vi "Configure Chevelle JESD Rx.vi"(0 "rx baseband session in":T1={"3630 session"={"VISA resource name"="", "Address Space"=1, "window_offset"=0, "register_addresses"={"MM based Registers"={"Revision"=0, "OldestCompatRev"=0, "signature"=0, "scratch"=0, "LedControl"=0, "BoardHwRev"=0, "BoardControl"=0, "ThermalStatus"=0, "BasebandStatus"=0, "BasebandControl"=0, "BasebandAuxSetup"=0, "BasebandAuxStatus"=0, "LmkSyncOutSetup"=0, " AdcSyncOutSetup"=0, " InjSyncOutSetup"=0, " PxiTrig0OutSetup"=0, " PxiTrig1OutSetup"=0, " PxiTrig2OutSetup"=0, " PxiTrig3OutSetup"=0, " PxiTrig4OutSetup"=0, " PxiTrig5OutSetup"=0, " PxiTrig6OutSetup"=0, " PxiTrig7OutSetup"=0}, "CPLD based Registers"={"SlaveSignature"=0, "SlaveRevision"=0, "SlaveOldestCompatRev"=0, "SlaveScratch"=0, "SlaveSetup"=0, "SlaveStatus"=0, "IDacReg_offset"=0, "LMKRegGrp0_offset"=0, "QDacReg_offset"=0, "BrdTempSensorVal"=0, "TempSensorPowerDown"=0, "GPIOReg_offset"=0, "IAdcReg_offset"=0, "QAdcReg_offset"=0, "LMKRegGrp1_offset"=0, "QadcTempSensorVal"=0, "IadcTempSensorVal"=0, "RevisionReg"=0, "VcxoReg"=0, "CpldStatusReg"=0, "PowerReg"=0, "VBiasEnReg"=0, "ExtRefOeReg"=0, "QdacCtrlReg"=0, "QdacStatusReg"=0, "IdacCtrlReg"=0, "IdacStatusReg"=0, "QdacJtagIn"=0, "QdacJtagOut"=0, "IdacJtagIn"=0, "IdacJtagOut"=0, "IqDcSetupReg"=0, "QadcStatusReg"=0, "IadcStatusReg"=0, "BrdSetupReg"=0, "IqDcRevisionReg"=0, "PllStatusReg"=0, "EndpointScratchReg"=0, "AdcSyncCfgReg"=0, "IqCardOpampReg"=0}, "CPLD Register Offset"=0, "MM  Register Offset"=0, " PxiTrig0OutSetup"=0}, "required_MM_fpga_version"={"signature"=0, "hardware"=0, "current revision"=0, "oldest revision"=0}, "CPLD Oldest Compat Version "={"hardware"=0, "CPLD firmware"=0}, "MM_FPGA_image_location"="", "is_init"=FALSE, "card_type"=enum."ADC", "DacLmkConfigFileName"="", "AdcLmkConfigFileName"="", "AdcConfigFileName"="", "DacConfigFileName_RevA"="", "DacConfigFileName_RevB"="", "Mulde hardware revision"=0, "bypass DAC PLL\n"=FALSE, "IQ Card Revision"=enum."RevA", "board capability"={"baseband sync"=enum."no baseband sync"}}, "7902 reference"=refnum} {"3630 session"."Address Space" items=["VXI/VME A16"=1, "VXI/VME A24"=2, "VXI/VME A32"=3, "VXI/VME A64"=4, "PXI Memory Allocations"=9, "PXI Configuration"=10, "PXI BAR0"=11, "PXI BAR1"=12, "PXI BAR2"=13, "PXI BAR3"=14, "PXI BAR4"=15, "PXI BAR5"=16]}, 11 "error in":errorcluster) -> (4 "rx baseband session":T1={"3630 session"={"VISA resource name"="", "Address Space"=1, "window_offset"=0, "register_addresses"={"MM based Registers"={"Revision"=0, "OldestCompatRev"=0, "signature"=0, "scratch"=0, "LedControl"=0, "BoardHwRev"=0, "BoardControl"=0, "ThermalStatus"=0, "BasebandStatus"=0, "BasebandControl"=0, "BasebandAuxSetup"=0, "BasebandAuxStatus"=0, "LmkSyncOutSetup"=0, " AdcSyncOutSetup"=0, " InjSyncOutSetup"=0, " PxiTrig0OutSetup"=0, " PxiTrig1OutSetup"=0, " PxiTrig2OutSetup"=0, " PxiTrig3OutSetup"=0, " PxiTrig4OutSetup"=0, " PxiTrig5OutSetup"=0, " PxiTrig6OutSetup"=0, " PxiTrig7OutSetup"=0}, "CPLD based Registers"={"SlaveSignature"=0, "SlaveRevision"=0, "SlaveOldestCompatRev"=0, "SlaveScratch"=0, "SlaveSetup"=0, "SlaveStatus"=0, "IDacReg_offset"=0, "LMKRegGrp0_offset"=0, "QDacReg_offset"=0, "BrdTempSensorVal"=0, "TempSensorPowerDown"=0, "GPIOReg_offset"=0, "IAdcReg_offset"=0, "QAdcReg_offset"=0, "LMKRegGrp1_offset"=0, "QadcTempSensorVal"=0, "IadcTempSensorVal"=0, "RevisionReg"=0, "VcxoReg"=0, "CpldStatusReg"=0, "PowerReg"=0, "VBiasEnReg"=0, "ExtRefOeReg"=0, "QdacCtrlReg"=0, "QdacStatusReg"=0, "IdacCtrlReg"=0, "IdacStatusReg"=0, "QdacJtagIn"=0, "QdacJtagOut"=0, "IdacJtagIn"=0, "IdacJtagOut"=0, "IqDcSetupReg"=0, "QadcStatusReg"=0, "IadcStatusReg"=0, "BrdSetupReg"=0, "IqDcRevisionReg"=0, "PllStatusReg"=0, "EndpointScratchReg"=0, "AdcSyncCfgReg"=0, "IqCardOpampReg"=0}, "CPLD Register Offset"=0, "MM  Register Offset"=0, " PxiTrig0OutSetup"=0}, "required_MM_fpga_version"={"signature"=0, "hardware"=0, "current revision"=0, "oldest revision"=0}, "CPLD Oldest Compat Version "={"hardware"=0, "CPLD firmware"=0}, "MM_FPGA_image_location"="", "is_init"=FALSE, "card_type"=enum."ADC", "DacLmkConfigFileName"="", "AdcLmkConfigFileName"="", "AdcConfigFileName"="", "DacConfigFileName_RevA"="", "DacConfigFileName_RevB"="", "Mulde hardware revision"=0, "bypass DAC PLL\n"=FALSE, "IQ Card Revision"=enum."RevA", "board capability"={"baseband sync"=enum."no baseband sync"}}, "7902 reference"=refnum} {"3630 session"."Address Space" items=["VXI/VME A16"=1, "VXI/VME A24"=2, "VXI/VME A32"=3, "VXI/VME A64"=4, "PXI Memory Allocations"=9, "PXI Configuration"=10, "PXI BAR0"=11, "PXI BAR1"=12, "PXI BAR2"=13, "PXI BAR3"=14, "PXI BAR4"=15, "PXI BAR5"=16]}, 15 "error out":errorcluster)   [LabVIEW 2019]
uses:
  TypeDefs/Rx Baseband Session.ctl
  <instrlib>/niMmWave/ni3610 and ni3630/controls/public/Main Settings.ctl
  <vilib>/Instr/_visa.llb/VISA Register Access Address Space.ctl
  <instrlib>/niMmWave/ni3610 and ni3630/controls/public/Register Adresses.ctl
  <instrlib>/niMmWave/ni3610 and ni3630/controls/public/Base Card Type.ctl
  <instrlib>/niMmWave/ni3610 and ni3630/controls/private/IQ Card Revision.ctl
  <instrlib>/niMmWave/ni3610 and ni3630/controls/public/Board Capability.ctl
  TypeDefs/Blank FPGA Reference.ctl
  TypeDefs/RX FPGA Reference.ctl
  <vilib>/rvi/errors/niLvFpgaAdjustHostInterfaceError.vi
  <vilib>/rvi/interface/nirviReadWriteControl/nirviReadWriteControl.xnode
  <vilib>/rvi/interface/Simulation/niFpgaSimulationCallBeginRW.vi
  NiFpgaLv.dll
  <instrlib>/niMmWave/ni3610 and ni3630/ni3610_and_ni3630_Driver_Lib.lvlib
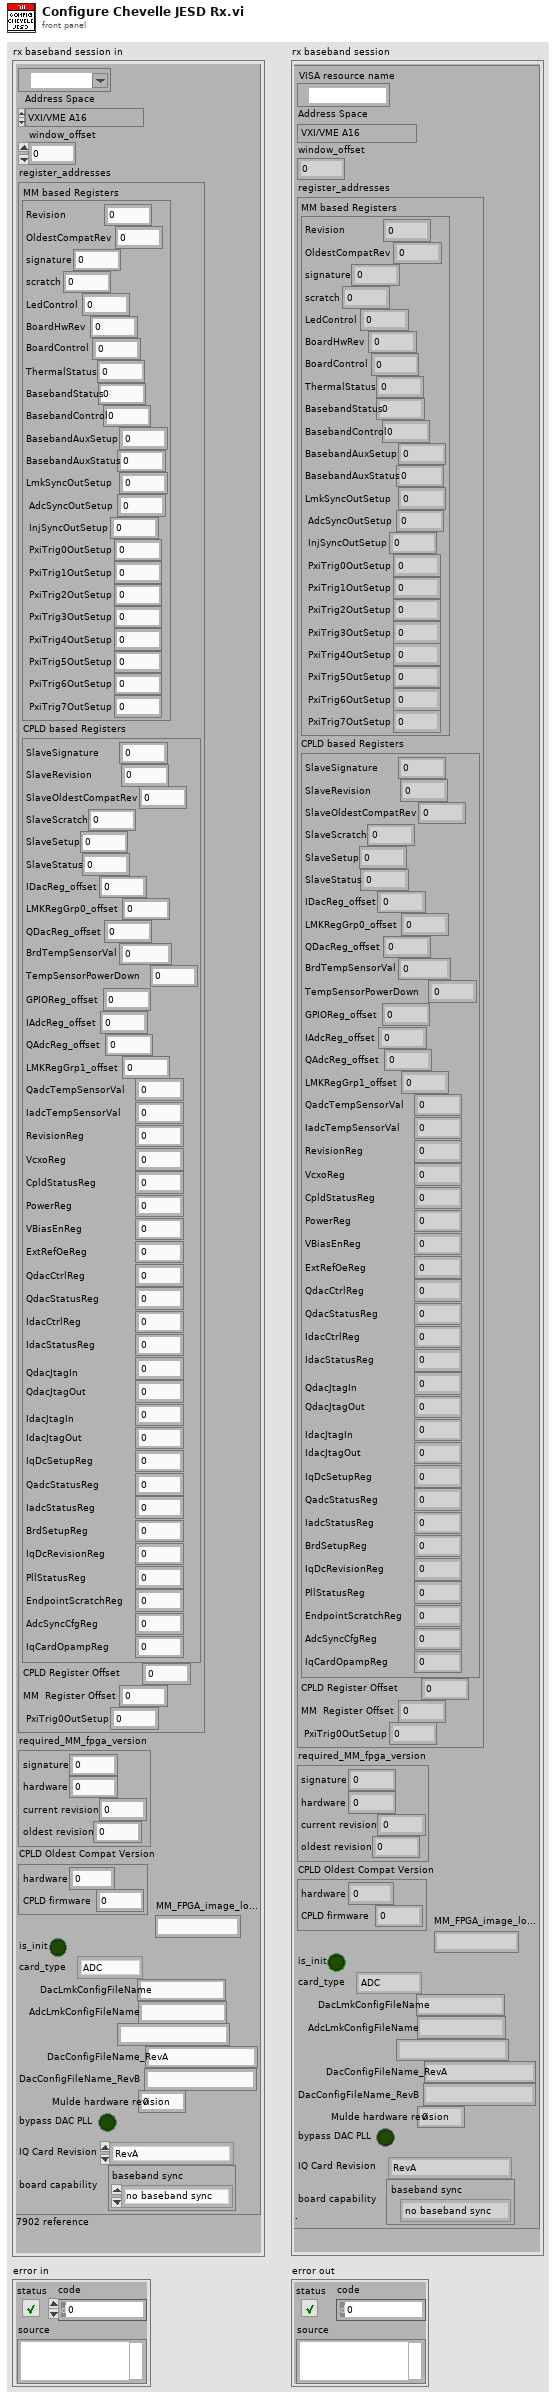
[diagram p1: front panel]
types:
  T1 = typedef "Rx Baseband Session.ctl" = cluster{"3630 session":T2, "7902 reference":T8}
  T2 = typedef "ni3610_and_ni3630_Driver_Lib.lvlib/Main Settings.ctl" = cluster{"VISA resource name":refnum<visa-resource-name>, "Address Space":T3, "window_offset":u32, "register_addresses":T4, "required_MM_fpga_version":cluster{"signature":u32, "hardware":u32, "current revision":u32, "oldest revision":u32}, "CPLD Oldest Compat Version ":cluster{"hardware":u32, "CPLD firmware":u32}, "MM_FPGA_image_location":string, "is_init":bool, "card_type":T5, "DacLmkConfigFileName":string, "AdcLmkConfigFileName":string, "AdcConfigFileName":string, "DacConfigFileName_RevA":string, "DacConfigFileName_RevB":string, "Mulde hardware revision":u8, "bypass DAC PLL\n":bool, "IQ Card Revision":T6, "board capability":T7}
  T3 = typedef "VISA Register Access Address Space.ctl" = u16
  T4 = typedef "ni3610_and_ni3630_Driver_Lib.lvlib/Register Adresses.ctl" = cluster{"MM based Registers":cluster{"Revision":u32, "OldestCompatRev":u32, "signature":u32, "scratch":u32, "LedControl":u32, "BoardHwRev":u32, "BoardControl":u32, "ThermalStatus":u32, "BasebandStatus":u32, "BasebandControl":u32, "BasebandAuxSetup":u32, "BasebandAuxStatus":u32, "LmkSyncOutSetup":u32, " AdcSyncOutSetup":u32, " InjSyncOutSetup":u32, " PxiTrig0OutSetup":u32, " PxiTrig1OutSetup":u32, " PxiTrig2OutSetup":u32, " PxiTrig3OutSetup":u32, " PxiTrig4OutSetup":u32, " PxiTrig5OutSetup":u32, " PxiTrig6OutSetup":u32, " PxiTrig7OutSetup":u32}, "CPLD based Registers":cluster{"SlaveSignature":u32, "SlaveRevision":u32, "SlaveOldestCompatRev":u32, "SlaveScratch":u32, "SlaveSetup":u32, "SlaveStatus":u32, "IDacReg_offset":u32, "LMKRegGrp0_offset":u32, "QDacReg_offset":u32, "BrdTempSensorVal":u32, "TempSensorPowerDown":u32, "GPIOReg_offset":u32, "IAdcReg_offset":u32, "QAdcReg_offset":u32, "LMKRegGrp1_offset":u32, "QadcTempSensorVal":u32, "IadcTempSensorVal":u32, "RevisionReg":u32, "VcxoReg":u32, "CpldStatusReg":u32, "PowerReg":u32, "VBiasEnReg":u32, "ExtRefOeReg":u32, "QdacCtrlReg":u32, "QdacStatusReg":u32, "IdacCtrlReg":u32, "IdacStatusReg":u32, "QdacJtagIn":u32, "QdacJtagOut":u32, "IdacJtagIn":u32, "IdacJtagOut":u32, "IqDcSetupReg":u32, "QadcStatusReg":u32, "IadcStatusReg":u32, "BrdSetupReg":u32, "IqDcRevisionReg":u32, "PllStatusReg":u32, "EndpointScratchReg":u32, "AdcSyncCfgReg":u32, "IqCardOpampReg":u32}, "CPLD Register Offset":u32, "MM  Register Offset":u32, " PxiTrig0OutSetup":u32}
  T5 = typedef "ni3610_and_ni3630_Driver_Lib.lvlib/Base Card Type.ctl" = enum16{"unspecified", "ADC", "DAC"}
  T6 = typedef "ni3610_and_ni3630_Driver_Lib.lvlib/IQ Card Revision.ctl" = enum16{"RevA", "RevB", "RevC", "RevD"}
  T7 = typedef "ni3610_and_ni3630_Driver_Lib.lvlib/Board Capability.ctl" = cluster{"baseband sync":enum16{"no baseband sync", "baseband sync"}}
  T8 = typedef "Blank FPGA Reference.ctl" = refnum<k20>
  T9 = typedef "RX FPGA Reference.ctl" = refnum<k20>
  T10 = cluster{"gtx active":bool, "jesd active":bool, "lane sync req":bool, "lanes synced":bool, "lanes aligned":bool, "qpll locked":bool, "qpll ref lost":bool, "k-char error":bool, "lane alignment error":bool, "8b10b error":bool, "8b10b disparity error":bool, "buffer overflow":bool, "buffer underflow":bool, "buffer ready":bool, "mgt ref clocks locked":bool, "mgt ref clock valid":bool, "config complete":bool}
  T11 = cluster{"gtx enable":bool, "jesd enable":bool, "sw sync":bool, "buffer enable":bool, "clock enable":bool, "trig5 output enable":bool, "trig5 invert":bool}
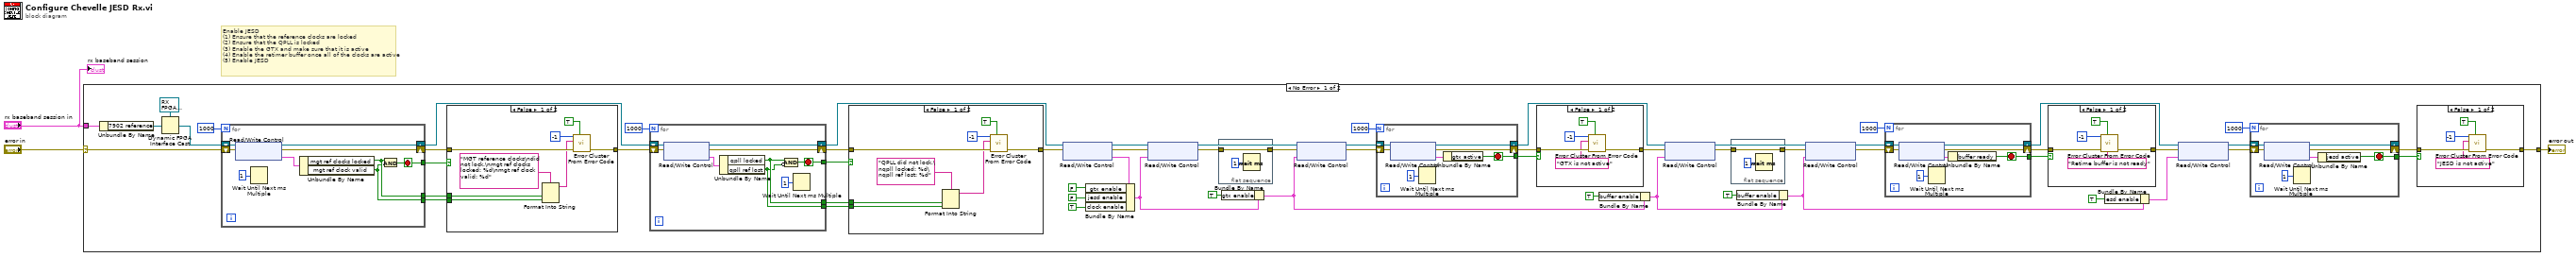
[diagram p0: block diagram]
diagram:
  # "Enable JESD\n(1) Ensure that the reference clocks are locked\n(2) Ensure that the QPLL is locked\n(3) Enable the GTX and make sure that it is active\n(4) Enable the retimer buffer once all of the clocks are active\n(5) Enable JESD"
  n1 = case shown="No Error" "error in" {
    selector: "error in" -> [w55 w143]
    tunnel: "rx baseband session in" -> [w34 _]
    tunnel: [w36 w143] -> w3
    frame No Error {
      n2 = Unbundle By Name(w34) -> ("7902 reference"=w35:T8)
      n3 = Dynamic FPGA Interface Cast(Session In=T9 refnum ("fpga reference"), Type=w35) -> (Session Out=w54:T9)
      n4 = for {
        N: 1000 -> [_]
        shift-right: [w76] -> w57
        shift-left: w54 -> [w74]
        shift-right: [w75] -> w59
        shift-left: w55 -> [w73]
        tunnel: [w71] -> w58
        tunnel: [w69] -> w7
        tunnel: [w68] -> w6
        stop <- w71 stop-if-true
        n5 = xnode "Read/Write Control"("FPGA VI Reference In"=w74, "error in"=w73) -> ("FPGA VI Reference Out"=w76:T9, "error out"=w75:errorcluster, "rxjesd.status"=w70:T10)
        n6 = Wait Until Next ms Multiple(millisecond multiple=u32 1) -> ()  [unwired: 1 out]
        n7 = Unbundle By Name(w70) -> ("mgt ref clocks locked"=w69:bool, "mgt ref clock valid"=w68:bool)
        n8 = Compound Arithmetic op=AND(w69, w68) -> (w71:bool)
      }
      n9 = case shown="False" w58 {
        tunnel: w59 -> [w84 w85]
        tunnel: [w83 w85] -> w56
        tunnel: w7 -> [w79 _]
        tunnel: w6 -> [w78 _]
        frame False {
          n10 = Format Into String(format string="MGT reference clocks\ndid not lock.\nmgt ref clocks locked: %d\nmgt ref clock valid: %d", w79, w78) -> (resulting string=w77:string)  [unwired: 2 in, 1 out]
          n11 = call <vilib>:"Error Cluster From Error Code.vi"("show call chain? (False)"=TRUE ("is warning? (False)"), "error in (no error)"=w84, "error message (\"\")"=w77, "error code (0)"=-1) -> ("error out"=w83:errorcluster)  [unwired: 5 in]
        }
        frame True {
        }
      }
      n12 = for {
        N: 1000 -> [_]
        shift-right: [w94] -> w12
        shift-left: w57 -> [w92]
        shift-right: [w93] -> w50
        shift-left: w56 -> [w91]
        tunnel: [w89] -> w51
        tunnel: [w87] -> w5
        tunnel: [w86] -> w4
        stop <- w89 stop-if-true
        n13 = xnode "Read/Write Control"("FPGA VI Reference In"=w92, "error in"=w91) -> ("FPGA VI Reference Out"=w94:T9, "error out"=w93:errorcluster, "rxjesd.status"=w88:T10)
        n14 = Unbundle By Name(w88) -> ("qpll locked"=w87:bool, "qpll ref lost"=w86:bool)
        n15 = Compound Arithmetic op=AND(w87, invert w86) -> (w89:bool)
        n16 = Wait Until Next ms Multiple(millisecond multiple=u32 1) -> ()  [unwired: 1 out]
      }
      n17 = case shown="False" w51 {
        tunnel: w50 -> [w102 w103]
        tunnel: [w101 w103] -> w13
        tunnel: w5 -> [w96 _]
        tunnel: w4 -> [w95 _]
        frame False {
          n18 = Format Into String(format string="QPLL did not lock.\nqpll locked: %d\nqpll ref lost: %d", w96, w95) -> (resulting string=w97:string)  [unwired: 2 in, 1 out]
          n19 = call <vilib>:"Error Cluster From Error Code.vi"("show call chain? (False)"=TRUE ("is warning? (False)"), "error in (no error)"=w102, "error message (\"\")"=w97, "error code (0)"=-1) -> ("error out"=w101:errorcluster)  [unwired: 5 in]
        }
        frame True {
        }
      }
      n20 = xnode "Read/Write Control"("FPGA VI Reference In"=w12, "error in"=w13) -> ("FPGA VI Reference Out"=w11:T9, "error out"=w14:errorcluster, "rxjesd.control"=w31:T11)
      n21 = Bundle By Name(cluster=w31, "gtx enable"=FALSE ("rxjesd.gtx enable"), "jesd enable"=FALSE ("rxjesd.jesd enable"), "clock enable"=TRUE ("clk enable")) -> (w17:T11)
      n22 = xnode "Read/Write Control"("FPGA VI Reference In"=w11, "error in"=w14, "rxjesd.control"=w17) -> ("FPGA VI Reference Out"=w53:T9, "error out"=w62:errorcluster)
      n23 = flat-sequence {
        tunnel: w62 -> [w66]
        tunnel: [w66] -> w52
        frame #0 {
          n24 = Wait (ms)(milliseconds to wait=u32 1) -> ()  [unwired: 1 out]
        }
      }
      n25 = Bundle By Name(cluster=w17, "gtx enable"=TRUE) -> (w8:T11)
      n26 = xnode "Read/Write Control"("FPGA VI Reference In"=w53, "error in"=w52, "rxjesd.control"=w8) -> ("FPGA VI Reference Out"=w47:T9, "error out"=w48:errorcluster)
      n27 = for {
        N: 1000 -> [_]
        shift-right: [w110] -> w33
        shift-left: w47 -> [w108]
        shift-right: [w109] -> w46
        shift-left: w48 -> [w107]
        tunnel: [w104] -> w45
        stop <- w104 stop-if-true
        n28 = xnode "Read/Write Control"("FPGA VI Reference In"=w108, "error in"=w107) -> ("FPGA VI Reference Out"=w110:T9, "error out"=w109:errorcluster, "rxjesd.status"=w105:T10)
        n29 = Wait Until Next ms Multiple(millisecond multiple=u32 1) -> ()  [unwired: 1 out]
        n30 = Unbundle By Name(w105) -> ("gtx active"=w104:bool)
      }
      n31 = case shown="False" w45 {
        tunnel: w46 -> [w115 w116]
        tunnel: [w114 w116] -> w32
        frame False {
          n32 = call <vilib>:"Error Cluster From Error Code.vi"("show call chain? (False)"=TRUE ("is warning? (False)"), "error in (no error)"=w115, "error message (\"\")"="GTX is not active" ("source"), "error code (0)"=-1) -> ("error out"=w114:errorcluster)  [unwired: 5 in]
        }
        frame True {
        }
      }
      n33 = Bundle By Name(cluster=w8, "buffer enable"=TRUE ("gtx enable")) -> (w16:T11)
      n34 = xnode "Read/Write Control"("FPGA VI Reference In"=w33, "error in"=w32, "rxjesd.control"=w16) -> ("FPGA VI Reference Out"=w22:T9, "error out"=w23:errorcluster)
      n35 = flat-sequence {
        tunnel: w23 -> [w64]
        tunnel: [w64] -> w19
        frame #0 {
          n36 = Wait (ms)(milliseconds to wait=u32 1) -> ()  [unwired: 1 out]
        }
      }
      n37 = Bundle By Name(cluster=w16, "buffer enable"=TRUE ("gtx enable")) -> (w15:T11)
      n38 = xnode "Read/Write Control"("FPGA VI Reference In"=w22, "error in"=w19, "rxjesd.control"=w15) -> ("FPGA VI Reference Out"=w21:T9, "error out"=w20:errorcluster)
      n39 = for {
        N: 1000 -> [_]
        shift-right: [w123] -> w10
        shift-left: w21 -> [w121]
        shift-right: [w122] -> w9
        shift-left: w20 -> [w120]
        tunnel: [w117] -> w43
        stop <- w117 stop-if-true
        n40 = xnode "Read/Write Control"("FPGA VI Reference In"=w121, "error in"=w120) -> ("FPGA VI Reference Out"=w123:T9, "error out"=w122:errorcluster, "rxjesd.status"=w118:T10)
        n41 = Wait Until Next ms Multiple(millisecond multiple=u32 1) -> ()  [unwired: 1 out]
        n42 = Unbundle By Name(w118) -> ("buffer ready"=w117:bool)
      }
      n43 = case shown="False" w43 {
        tunnel: w9 -> [w128 w129]
        tunnel: [w127 w129] -> w42
        frame False {
          n44 = call <vilib>:"Error Cluster From Error Code.vi"("show call chain? (False)"=TRUE ("is warning? (False)"), "error in (no error)"=w128, "error message (\"\")"="Retime buffer is not ready" ("source"), "error code (0)"=-1) -> ("error out"=w127:errorcluster)  [unwired: 5 in]
        }
        frame True {
        }
      }
      n45 = Bundle By Name(cluster=w15, "jesd enable"=TRUE ("gtx enable")) -> (w24:T11)
      n46 = xnode "Read/Write Control"("FPGA VI Reference In"=w10, "error in"=w42, "rxjesd.control"=w24) -> ("FPGA VI Reference Out"=w38:T9, "error out"=w37:errorcluster)
      n47 = for {
        N: 1000 -> [_]
        shift-right: [w136] -> _
        shift-left: w38 -> [w134]
        shift-right: [w135] -> w40
        shift-left: w37 -> [w133]
        tunnel: [w130] -> w39
        stop <- w130 stop-if-true
        n48 = xnode "Read/Write Control"("FPGA VI Reference In"=w134, "error in"=w133) -> ("FPGA VI Reference Out"=w136:T9, "error out"=w135:errorcluster, "rxjesd.status"=w131:T10)
        n49 = Wait Until Next ms Multiple(millisecond multiple=u32 1) -> ()  [unwired: 1 out]
        n50 = Unbundle By Name(w131) -> ("jesd active"=w130:bool)
      }
      n51 = case shown="False" w39 {
        tunnel: w40 -> [w141 w142]
        tunnel: [w140 w142] -> w36
        frame False {
          n52 = call <vilib>:"Error Cluster From Error Code.vi"("show call chain? (False)"=TRUE ("is warning? (False)"), "error in (no error)"=w141, "error message (\"\")"="JESD is not active" ("source"), "error code (0)"=-1) -> ("error out"=w140:errorcluster)  [unwired: 5 in]
        }
        frame True {
        }
      }
    }
    frame Error {
    }
  }
  "error out" <- w3
  "rx baseband session" <- "rx baseband session in"
